vi "QTrkFinalizeLUT.vi"(4 "error in (no error)":errorcluster, 7 "QTrk Instance":T1) -> (0 "error out":errorcluster, 3 "QTrk Instance":T1)   [LabVIEW 2011]
uses:
  QTrkInstance.ctl
  QTrkDLL.vi
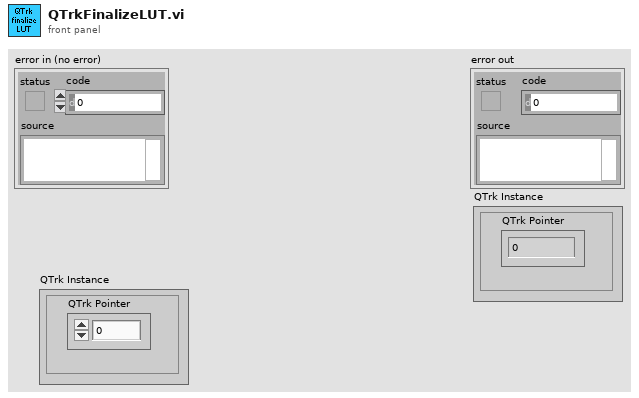
[diagram p1: front panel]
types:
  T1 = typedef "QTrkInstance.ctl" = cluster{"QTrk Pointer":u64}
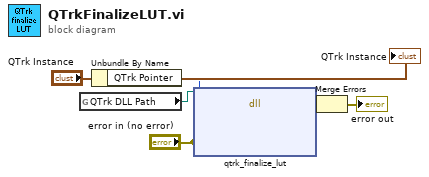
[diagram p0: block diagram]
diagram:
  n1 = global read "QTrkDLL.vi" "QTrk DLL Path"() -> (w7:path)
  n2 = Unbundle By Name("QTrk Instance") -> ("QTrk Pointer"=w5:u64)
  n3 = dll-call lib="D:/jcnossen1/cudaqi-tracker/cudatrack-labview/cputrack_d.dll" fn="qtrk_finalize_lut"(path in=w7, error in="error in (no error)", "tracker"=w5, "error"="error in (no error)") -> (error out=w3:errorcluster, "error"=w2:errorcluster)  [unwired: 3 in, 1 out]
  n4 = Merge Errors(w3, w2) -> (→"error out":errorcluster)
  "QTrk Instance" <- "QTrk Instance"
